vi "server.Format Client Request (Notification).vi"(8 "error in (no error)":errorcluster, 9 "id":string, 10 "JSON in":refnum<class "JSON Null.lvclass">, 11 "method":string) -> (0 "error out":errorcluster, 2 "Request String":string)   [LabVIEW 2016, in "JSONRPC Server.lvclass"]
uses:
  JSONRPC Server.lvclass
  <vilib>/NI/JSON Support for LabVIEW/JSON Data Classes/JSON Datatype/JSON Null.lvclass
  <vilib>/NI/JSON Support for LabVIEW/JSON Data Classes/JSON Object/JSON Object.lvclass
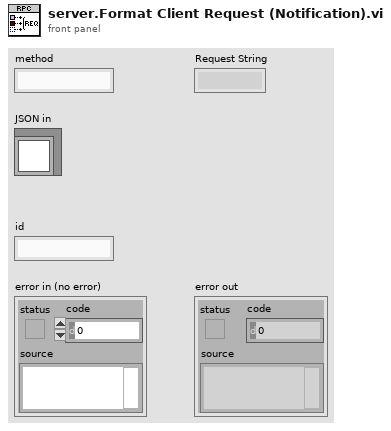
[diagram p1: front panel]
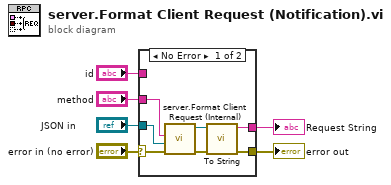
[diagram p0: block diagram]
diagram:
  n1 = case shown="No Error" "error in (no error)" {
    selector: "error in (no error)" -> [w13 w14]
    tunnel: [w12 w14] -> w5
    tunnel: "JSON in" -> [w7 _]
    tunnel: [w11 _] -> w3
    tunnel: "method" -> [w10 _]
    tunnel: "id" -> [_ _]
    frame No Error {
      n2 = call "server.Format Client Request (Internal).vi"("error in (no error)"=w13, "params"=w7, "method"=w10) -> ("error out"=w9:errorcluster, "JSON Object out"=w8:refnum<class "JSON Object.lvclass">)  [unwired: 7 in]
      n3 = call-dynamic "To String.vi"("error in (no error)"=w9, "JSON Object in"=w8) -> ("error out"=w12:errorcluster, "String"=w11:string)  [unwired: 8 in]
    }
    frame Error {
    }
  }
  "error out" <- w5
  "Request String" <- w3
